vi "Write conversion file.vi"(8 "error in (no error)":errorcluster, 11 "DAQOrcaFlash in":refnum<class "DAQOrcaFlash.lvclass">) -> (0 "error out":errorcluster, 3 "DAQOrcaFlash out":refnum<class "DAQOrcaFlash.lvclass">)   [LabVIEW 2012, in "DAQOrcaFlash.lvclass"]
uses:
  DAQOrcaFlash.lvclass
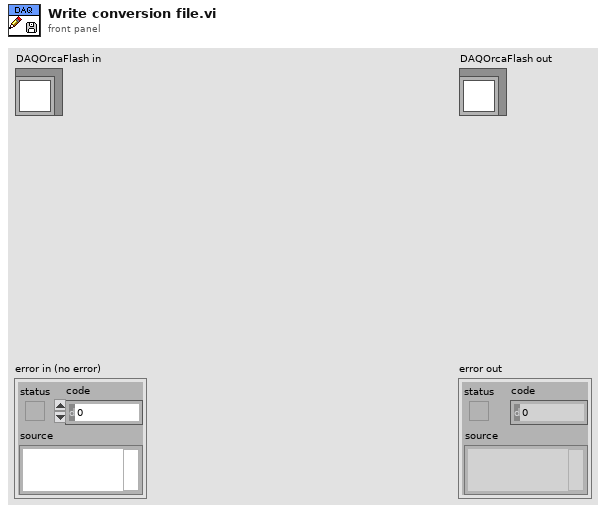
[diagram p1: front panel]
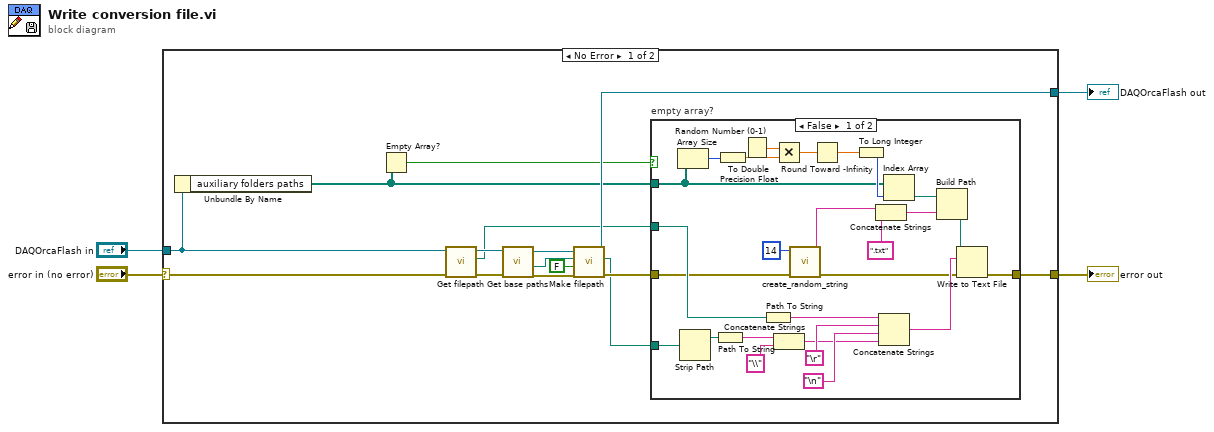
[diagram p0: block diagram]
diagram:
  n1 = case shown="No Error" "error in (no error)" {
    selector: "error in (no error)" -> [w12 w48]
    tunnel: [w18 w48] -> w3
    tunnel: [w17 w47] -> w1
    tunnel: "DAQOrcaFlash in" -> [w5 w47]
    frame No Error {
      n2 = Unbundle By Name(w5) -> ("auxiliary folders paths"=w7:path[])
      n3 = Empty Array?(array=w7) -> (empty?=w6:bool)
      n4 = call "Get filepath.vi"("error in (no error)"=w12, "DAQOrcaFlash in"=w5) -> ("error out"=w11:errorcluster, "full storage path"=w9:path, "DAQOrcaFlash out"=w10:refnum<class "DAQOrcaFlash.lvclass">)  [unwired: 7 in]
      n5 = call-dynamic "Get base paths.vi"("error in (no error)"=w11, "DAQOrcaFlash in"=w10) -> ("error out"=w14:errorcluster, "final conversion folder"=w16:path, "DAQOrcaFlash out"=w13:refnum<class "DAQOrcaFlash.lvclass">)  [unwired: 6 in, 1 out]
      n6 = call "Make filepath.vi"("error in (no error)"=w14, "is cxd file path?"=FALSE, "base path"=w16, "DAQOrcaFlash in"=w13) -> ("error out"=w19:errorcluster, "filepath out"=w15:path, "DAQOrcaFlash out"=w17:refnum<class "DAQOrcaFlash.lvclass">)  [unwired: 5 in]
      n7 = case "empty array?" shown="False" w6 {
        tunnel: w19 -> [w25 w46]
        tunnel: [w39 w46] -> w18
        tunnel: w9 -> [w38 _]
        tunnel: w7 -> [w27 _]
        tunnel: w15 -> [w37 _]
        frame False {
          n8 = Array Size(array=w27) -> (size(s)=w31:i32)
          n9 = Strip Path(path=w37) -> (stripped path=w45:path)  [unwired: 1 out]
          n10 = Path To String(path=w45) -> (string=w35:string)
          n11 = To Double Precision Float(number=w31) -> (double precision float=w32:dbl)
          n12 = Random Number (0-1)() -> (number: 0 to 1=w33:dbl)
          n13 = Path To String(path=w38) -> (string=w42:string)
          n14 = Multiply(x=w33, y=w32) -> (x*y=w30:dbl)
          n15 = Concatenate Strings(w35, "\\" ("string")) -> (w36:string)
          n16 = call "create_random_string.vi"("error in (no error)"=w25, "length"=14) -> ("error out"=w20:errorcluster, "random string"=w22:string)  [unwired: 8 in]
          n17 = Round Toward -Infinity(1:w30) -> (0:w29:dbl)
          n18 = To Long Integer(number=w29) -> (32bit integer=w28:i32)
          n19 = Concatenate Strings(w22, ".txt" ("format string")) -> (w21:string)
          n20 = Concatenate Strings(w42, "\r", "\n", w36) -> (w40:string)
          n21 = Index Array(array=w27, index=w28) -> (element=w26:path)
          n22 = Build Path(base path=w26, name or relative path=w21) -> (appended path=w41:path)
          n23 = Write to Text File(file (use dialog)=w41, text=w40, error in=w20) -> (error out=w39:errorcluster)  [unwired: 1 in, 2 out]
        }
        frame True {
        }
      }
    }
    frame Error {
    }
  }
  "error out" <- w3
  "DAQOrcaFlash out" <- w1
